vi "Get ByVal.vi"(8 "error in (no error)":errorcluster, 11 "Numeric in":refnum<class "Numeric Test Object.lvclass">) -> (0 "error out":errorcluster, 2 "Int":i32, 3 "Numeric out":refnum<class "Numeric Test Object.lvclass">)   [LabVIEW 2009, in "Numeric Test Object.lvclass"]
uses:
  Numeric Test Object.lvclass
  Numeric Test Object.lvclass/Numeric Test Object.ctl
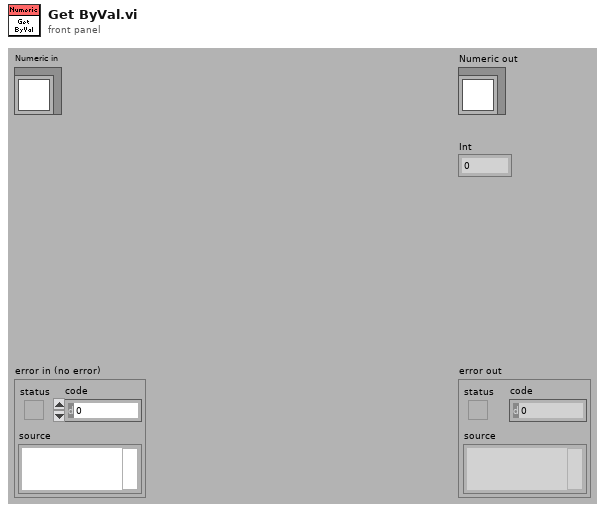
[diagram p1: front panel]
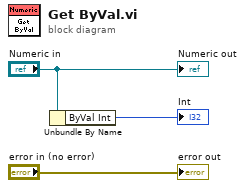
[diagram p0: block diagram]
diagram:
  n1 = Unbundle By Name("Numeric in") -> ("ByVal Int"=→"Int":i32)
  "error out" <- "error in (no error)"
  "Numeric out" <- "Numeric in"
